vi "NicmosGetTemperature.vi"(9 "error in (no error)":errorcluster caption="error out (no error)") -> (2 "Graphe déroulant":cluster{"T1":dbl, "T2":dbl}(graph), 6 "error out":errorcluster)   [LabVIEW 2009]
uses:
  Controls/NICMOS.COMMAND.ctl
  Controls/NICMOS.COMMANDBASIC.ctl
  Controls/NICMOS.READOUT.ctl
  Controls/NICMOS.FILTERCOMMAND.ctl
  Controls/NICMOS.FILTER.ctl
  Controls/NICMOS.TEMPERATURE.ctl
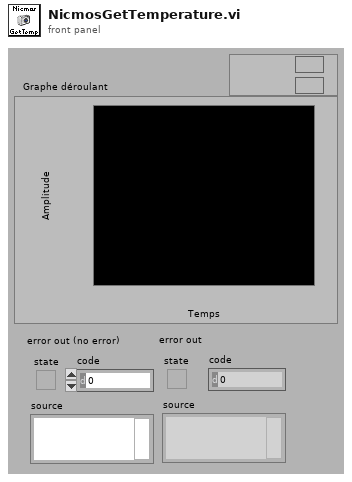
[diagram p1: front panel]
types:
  T1 = typedef "NICMOS.TEMPERATURE.ctl" = cluster{"T1":dbl, "T2":dbl}
  T2 = typedef "NICMOS.COMMAND.ctl" = cluster{"Command":T3, "READOUT":T4, "FILTERCOMMAND":T5, "ACQUISITION":i32, "Done":refnum<k4>}
  T3 = typedef "NICMOS.COMMANDBASIC.ctl" = enum16{"WRITE BANKS", "SET FILTER", "HOME FILTER", "QUERY TEMP", "CONFIGURE", "START", "ACQUISITION", "STOP", "QUIT"}
  T4 = typedef "NICMOS.READOUT.ctl" = cluster{"Readout":i32, "Deglitch":i32, "Framerate":dbl[unit], "Bank":i32}
  T5 = typedef "NICMOS.FILTERCOMMAND.ctl" = cluster{"FILTER":T6, "INIT":bool}
  T6 = typedef "NICMOS.FILTER.ctl" = string
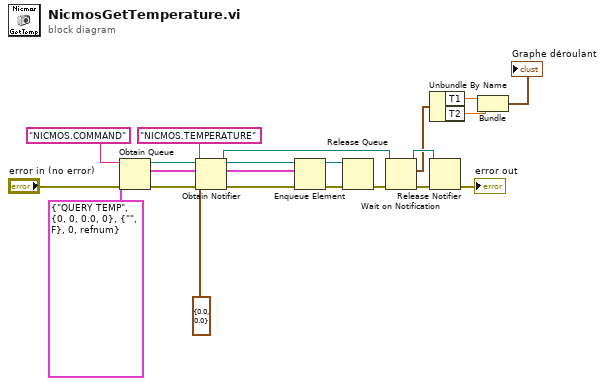
[diagram p0: block diagram]
diagram:
  w7 = T2 {"Command"=enum."QUERY TEMP", "READOUT"={"Readout"=0, "Deglitch"=0, "Framerate"=0.0, "Bank"=0}, "FILTERCOMMAND"={"FILTER"="", "INIT"=FALSE}, "ACQUISITION"=0, "Done"=refnum} ("NicmosCommand")
  n1 = Obtain Queue(name (unnamed)="NICMOS.COMMAND" ("nom (aucun)"), element data type=w7, error in (no error)="error in (no error)") -> (queue out=w5:refnum<queue>, error out=w16:errorcluster)  [unwired: 2 in, 1 out]
  n2 = Obtain Notifier(name (unnamed)="NICMOS.TEMPERATURE" ("nom (aucun)"), notification data type=T1 {"T1"=0.0, "T2"=0.0} ("Nicmos Status"), error in (no error)=w16) -> (notifier out=w3:refnum<notifier>, error out=w15:errorcluster)  [unwired: 1 in, 1 out]
  n3 = Enqueue Element(queue=w5, element=w7, error in (no error)=w15) -> (queue out=w4:refnum<queue>, error out=w18:errorcluster)  [unwired: 1 in, 1 out]
  n4 = Release Queue(queue=w4, error in (no error)=w18) -> (error out=w6:errorcluster)  [unwired: 1 in, 2 out]
  n5 = Wait on Notification(notifier=w3, error in (no error)=w6) -> (notifier out=w2:refnum<notifier>, notification=w1:T1, error out=w11:errorcluster)  [unwired: 2 in, 1 out]
  n6 = Unbundle By Name(w1) -> ("T1"=w10:dbl, "T2"=w9:dbl)
  n7 = Release Notifier(notifier=w2, error in (no error)=w11) -> (error out=→"error out":errorcluster)  [unwired: 1 in, 2 out]
  n8 = Bundle("T1"=w10, "T2"=w9) -> (→"Graphe déroulant":cluster{"T1":dbl, "T2":dbl})  [unwired: 1 in]
